vi "Set Flow Capacity Unit--SubVI.vi"(8 "error in (no error)":errorcluster, 9 "Standard Volume Flow":T1 items=["uls/h", "uls/min", "uls/s", "mls/h", "mls/min", "mls/s", "ls/h", "ls/min", "ls/s", "ccs/h", "ccn/min", "ccs/s", "mm3s/h", "mm3s/m", "mm3s/s", "cm3s/h", "cm3s/m", "cm3s/s", "m3s/h", "m3s/min", "m3s/s"], 10 "Device":T10, 11 "Data Cluster":T2 {"Flexi-Flow Devices"."Control State"."Control Mode" items=["Bus/RS232"=0, "FLOW-BUS slave"=2, "Valve close"=3, "Controller idle"=4, "Setpoint 100%"=7, "Valve fully open"=8, "Calibration mode"=9, "Setpoint 0%"=12, "RS232"=18, "Valve steering"=20, "Valve safe state"=22]}) -> (0 "error out":errorcluster, 2 "Value":string, 3 "Data Cluster Out":T2 {"Flexi-Flow Devices"."Control State"."Control Mode" items=["Bus/RS232"=0, "FLOW-BUS slave"=2, "Valve close"=3, "Controller idle"=4, "Setpoint 100%"=7, "Valve fully open"=8, "Calibration mode"=9, "Setpoint 0%"=12, "RS232"=18, "Valve steering"=20, "Valve safe state"=22]})   [LabVIEW 2024, in "FlexiFlowInterfaceCH2.lvlib"]
uses:
  FlexiFlowInterfaceCH2.lvlib
  FlexiFlowDevice--enum.ctl
  Module Data--cluster.ctl
  Modbus TCP Connection Settings--cluster.ctl
  Modbus Flexi-Flow State--cluster.ctl
  <vilib>/Plasmionique/MB Master/MB_Master_TCP/MB_Master_TCP.lvclass
  Device Type--enum.ctl
  Modbus Flexi-Flow Controls--cluster.ctl
  Modbus Flexi-Flow API/Control Mode--enum.ctl
  Modbus Flexi-Flow API/Control Function Values--enum.ctl
  Modbus Flexi-Flow Measure State--cluster.ctl
  Modbus Flexi-Flow API/Capacity Units (Standard Volume Flow).ctl
  Modbus Flexi-Flow API/PDU Address String Params--ring.ctl
  Modbus Flexi-Flow API/Write String Register.vi
  Modbus Flexi-Flow API/Read String Register.vi
  Modbus Flexi-Flow API/Bronkhorst Flexi-Flow ModbusTCP API.lvlib
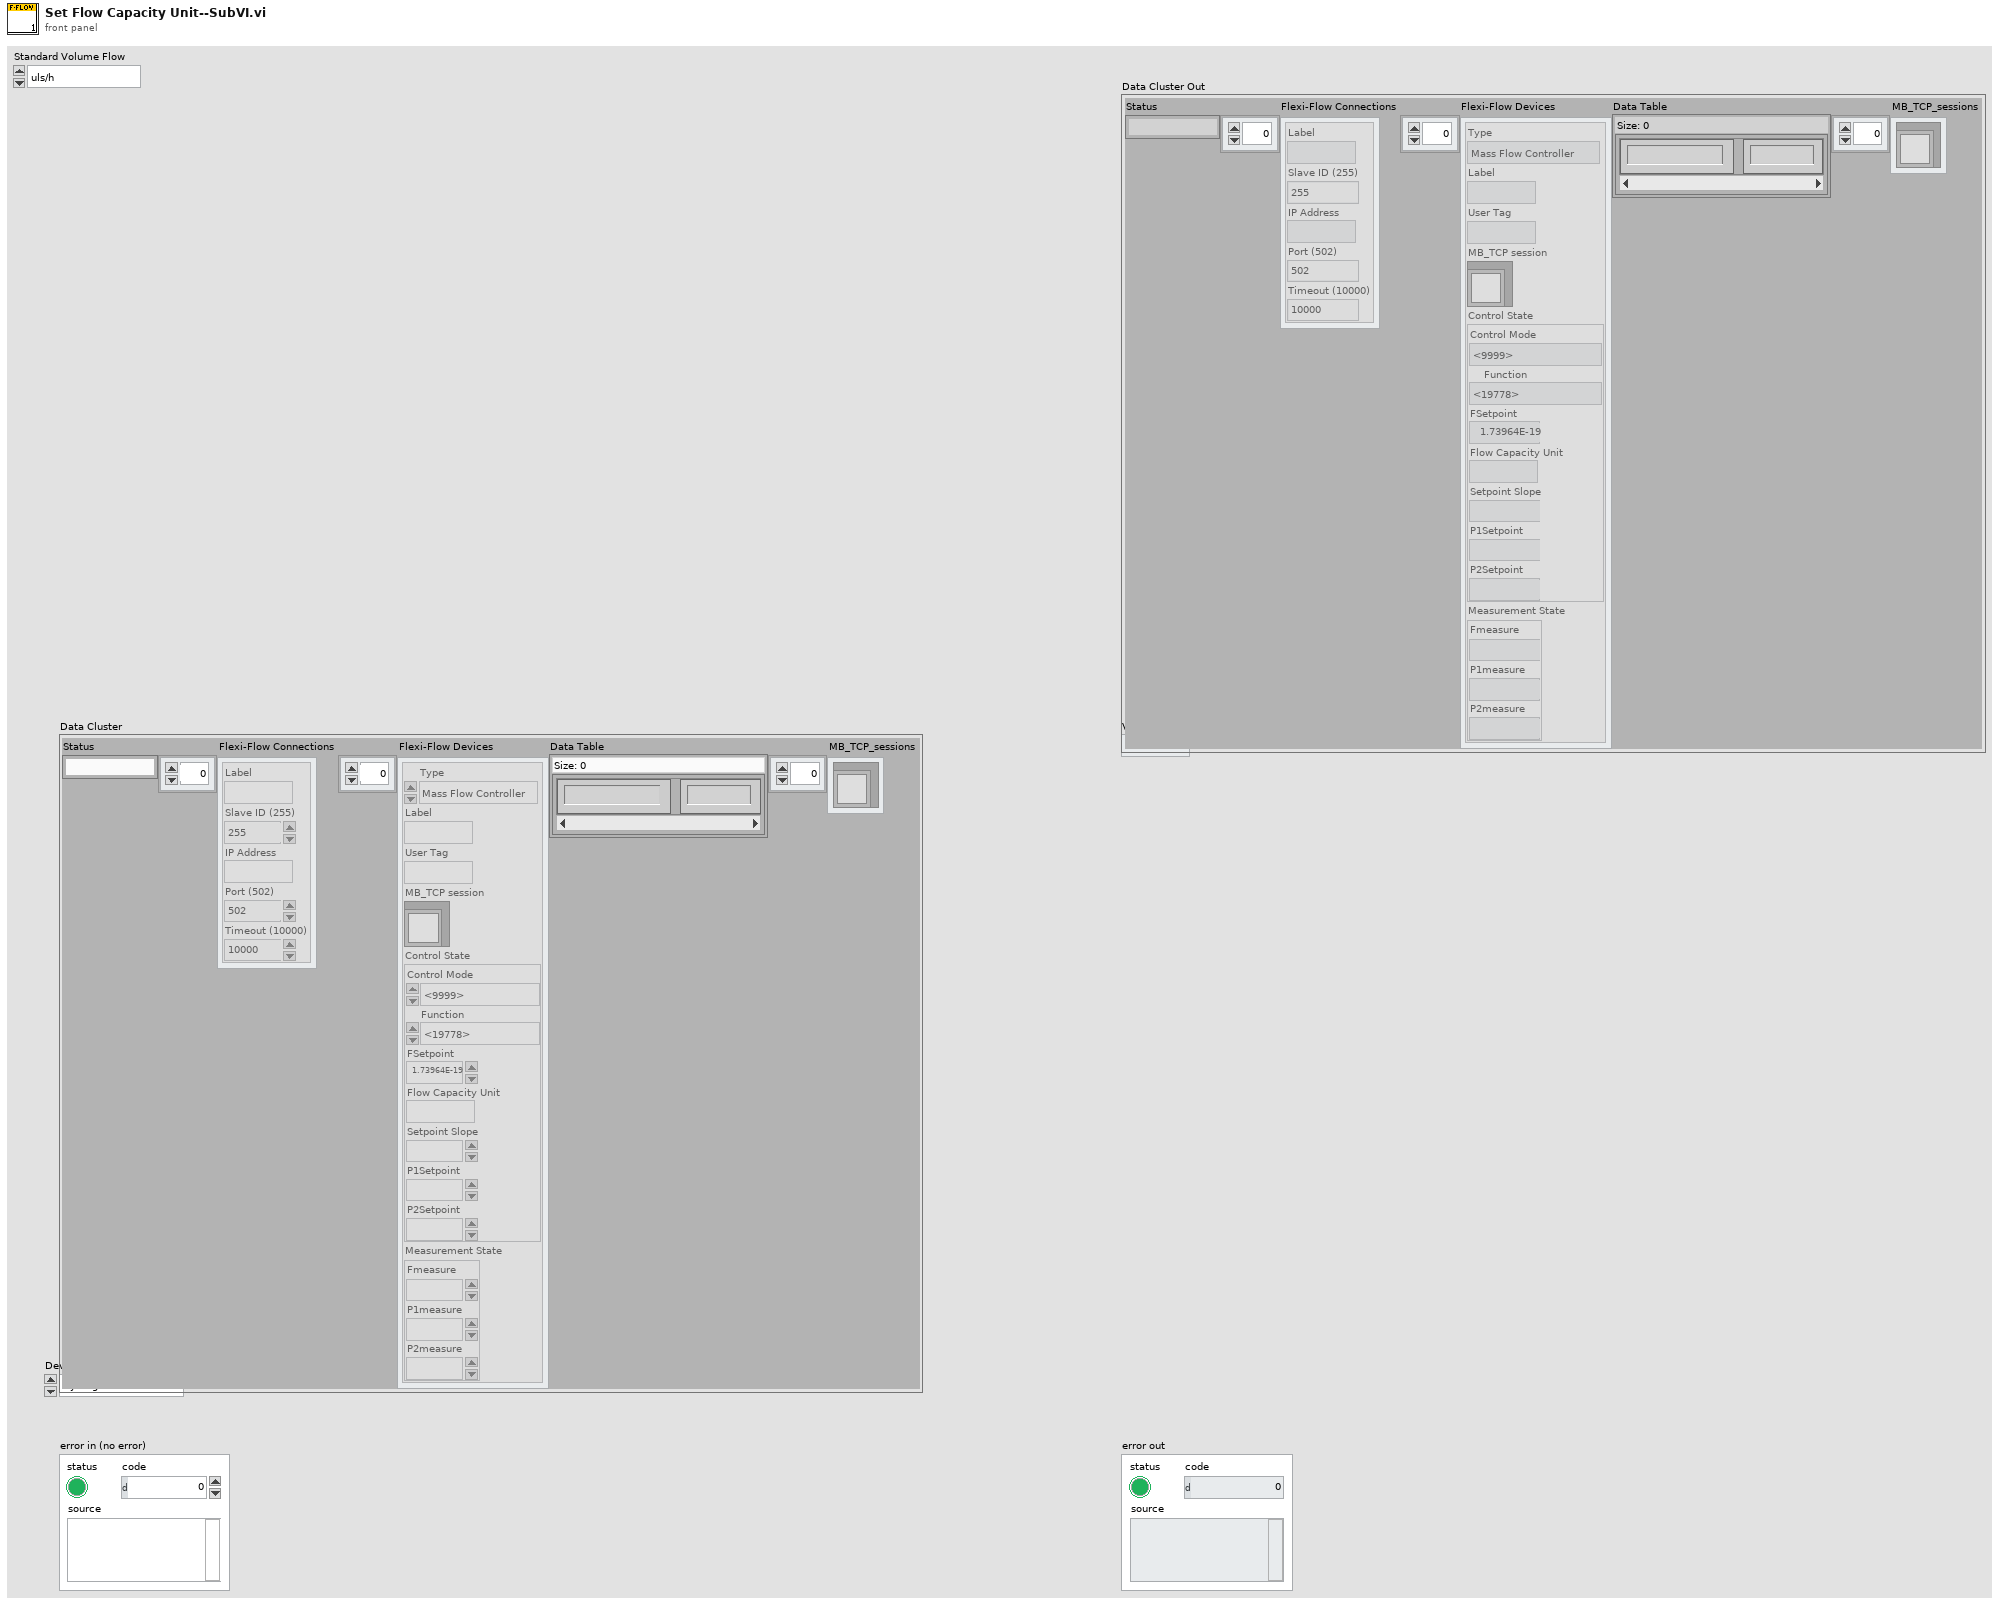
[diagram p1: front panel]
types:
  T1 = typedef "Bronkhorst Flexi-Flow ModbusTCP API.lvlib/Capacity Units (Standard Volume Flow).ctl" = u16
  T2 = typedef "FlexiFlowInterfaceCH2.lvlib/Module Data--cluster.ctl" = cluster{"Status":string, "Flexi-Flow Connections":T3[], "Flexi-Flow Devices":T4[], "Data Table":map{string, dbl}, "MB_TCP_sessions":refnum<class "MB_Master_TCP.lvclass">[]}
  T3 = typedef "FlexiFlowInterfaceCH2.lvlib/Modbus TCP Connection Settings--cluster.ctl" = cluster{"Label":string, "Slave ID (255)":u8, "IP Address":string, "Port (502)":u16, "Timeout (10000)":i32}
  T4 = typedef "FlexiFlowInterfaceCH2.lvlib/Modbus Flexi-Flow State--cluster.ctl" = cluster{"Type":T5, "Label":string, "User Tag":string, "MB_TCP session":refnum<class "MB_Master_TCP.lvclass">, "Control State":T6, "Measurement State":T9}
  T5 = typedef "FlexiFlowInterfaceCH2.lvlib/Device Type--enum.ctl" = enum16{"Mass Flow Controller", "Mass Flow Meter"}
  T6 = typedef "FlexiFlowInterfaceCH2.lvlib/Modbus Flexi-Flow Controls--cluster.ctl" = cluster{"Control Mode":T7, "Function":T8, "FSetpoint":sgl, "Flow Capacity Unit":string, "Setpoint Slope":u16, "P1Setpoint":sgl, "P2Setpoint":sgl}
  T7 = typedef "Bronkhorst Flexi-Flow ModbusTCP API.lvlib/Control Mode--enum.ctl" = u16
  T8 = typedef "Bronkhorst Flexi-Flow ModbusTCP API.lvlib/Control Function Values--enum.ctl" = enum16{"Flow", "Upstream pressure", "Downstream pressure", "Flow with upstream pressure limit", "Flow with downstream pressure limit", "Upstream pressure with flow limit", "Downstream pressure with flow limit"}
  T9 = typedef "FlexiFlowInterfaceCH2.lvlib/Modbus Flexi-Flow Measure State--cluster.ctl" = cluster{"Fmeasure":dbl, "P1measure":sgl, "P2measure":sgl}
  T10 = typedef "FlexiFlowInterfaceCH2.lvlib/FlexiFlowDevice--enum.ctl" = enum16{"Hydrogen Inlet", "Nitrogen Inlet", "Cathode Outlet", "Anode Outlet"}
  T11 = typedef "Bronkhorst Flexi-Flow ModbusTCP API.lvlib/PDU Address String Params--ring.ctl" = u16
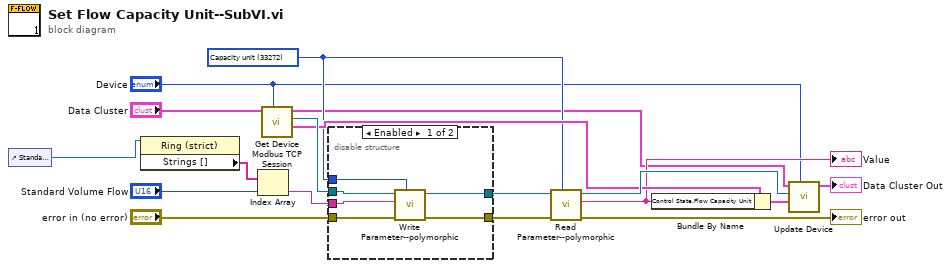
[diagram p0: block diagram]
diagram:
  w12 = T11 33272 items=["Fluid name"=33160, "Capacity unit"=33272, "User tag"=61744] ("PDU Address String Params")
  n1 = control-ref of="Standard Volume Flow"() -> (w2:refnum<vi>)
  n2 = property class="Ring (strict)"(reference=w2) -> ("Strings []"=w13:string[])  [unwired: 1 in, 2 out]
  n3 = Index Array(array=w13, index="Standard Volume Flow") -> (element=w14:string)
  n4 = call "Get Device Modbus TCP Session.vi"("Device"="Device", "Data Cluster In"="Data Cluster") -> ("Device State"=w15:T4, "MB_TCP session"=w18:refnum<class "MB_Master_TCP.lvclass">, "Data Cluster Out"=w4:T2)  [unwired: 7 in]
  n5 = disable-structure shown="Enabled" {
    disable-tunnel: "error in (no error)" -> [w24 w26]
    disable-tunnel: [w23 w26] -> w8
    disable-tunnel: w18 -> [w22 w25]
    disable-tunnel: [w21 w25] -> w9
    disable-tunnel: w12 -> [w20 _]
    disable-tunnel: w14 -> [w19 _]
    frame Enabled {
      n6 = call-poly "Write Parameter--polymorphic.vi"("PDU Address String Params"=w20, "error in"=w24, "String"=w19, "MB_TCP session in"=w22) -> ("error out"=w23:errorcluster, "MB session out"=w21:refnum<class "MB_Master_TCP.lvclass">)  [unwired: 6 in]
    }
    frame Disabled {
    }
  }
  n7 = call-poly "Read Parameter--polymorphic.vi"("PDU Address String Params"=w12, "error in"=w8, "MB_TCP session in"=w9) -> ("error out"=→"error out":errorcluster, "Value"=w11:string, "MB session out"=w17:refnum<class "MB_Master_TCP.lvclass">)  [unwired: 6 in]
  "Value" <- w11
  n8 = Bundle By Name(cluster=w15, "Control State.Flow Capacity Unit"=w11) -> (w16:T4)
  n9 = call "Update Device.vi"("Device"="Device", "Device State"=w16, "MB_TCP session"=w17, "Data Cluster"=w4) -> ("Data Cluster Out"=→"Data Cluster Out":T2)  [unwired: 7 in]
